vi "Homing RIO.vi"(7 "Offset Home 2 RCM":dbl[](array[numeric])=[0.0, 0.0, 0.0, 0.0], 8 "error in":errorcluster, 9 "Stage PID Cluster":T2={"Stage Z PID"={"Kp"=0.0005, "Kd"=0.001, "Ki"=0.0}, "Stage Y PID"={"Kp"=0.0003, "Kd"=0.01, "Ki"=0.0}, "Stage X PID"={"Kp"=0.0003, "Kd"=0.01, "Ki"=0.0}}, 10 "L1 to L4 PID Cluster":T1={"L1 PID Gains"={"Kp"=0.005, "Kd"=0.5, "Ki"=0.0005}, "L2 PID Gains"={"Kp"=0.01, "Kd"=1.0, "Ki"=0.005}, "L3 PID Gains"={"Kp"=0.05, "Kd"=1.0, "Ki"=0.0005}, "L4 PID Gains"={"Kp"=0.1, "Kd"=0.1, "Ki"=0.0005}}, 11 "FPGA VI Reference In":refnum<k20>) -> (0 "error out":errorcluster, 1 "Last Stage Posit":dbl[](array[numeric]), 2 "Last L1 to L4 Posit":dbl[](array[numeric]), 3 "FPGA VI Reference Out":refnum<k20>)   [LabVIEW 2016]
uses:
  <vilib>/Platform/TimedLoop/XDataNode/timing_clust.ctl
  <vilib>/Platform/TimedLoop/XDataNode/nitl_modes.ctl
  <vilib>/Platform/TimedLoop/XDataNode/wakeup.ctl
  Library/KevinLibraryAll/labview2010/kevLib2010/Simple Filters/kDelay.vi
  Global Variables.vi
  <vilib>/Utility/error.llb/Error Cluster From Error Code.vi
  <vilib>/rvi/errors/niLvFpgaAdjustHostInterfaceError.vi
  <vilib>/platform/TimedLoop/XDataNode/XDataNode.xnode
  <vilib>/rvi/interface/nirviReadWriteControl/nirviReadWriteControl.xnode
  FPGA Bitfiles/IRISSTrack_FPGATarget2_IRISSFPGAIORIO_4NTO9ubhv-c.lvbitx
  IRISS_FPGA_IO_RIO.vi
  <vilib>/Platform/TimedLoop/XDataNode/XDNodeRunTimeDep.lvlib
  Library/KevinLibraryAll/labview2010/kevLib2010.lvlib
  Library/KevinLibraryAll/labview2011/kevLib2011.lvlib
  Library/KevinLibraryAll/labview/KevLib01.lvlib
  Library/jmslib.lvlib
  NiFpgaLv.dll
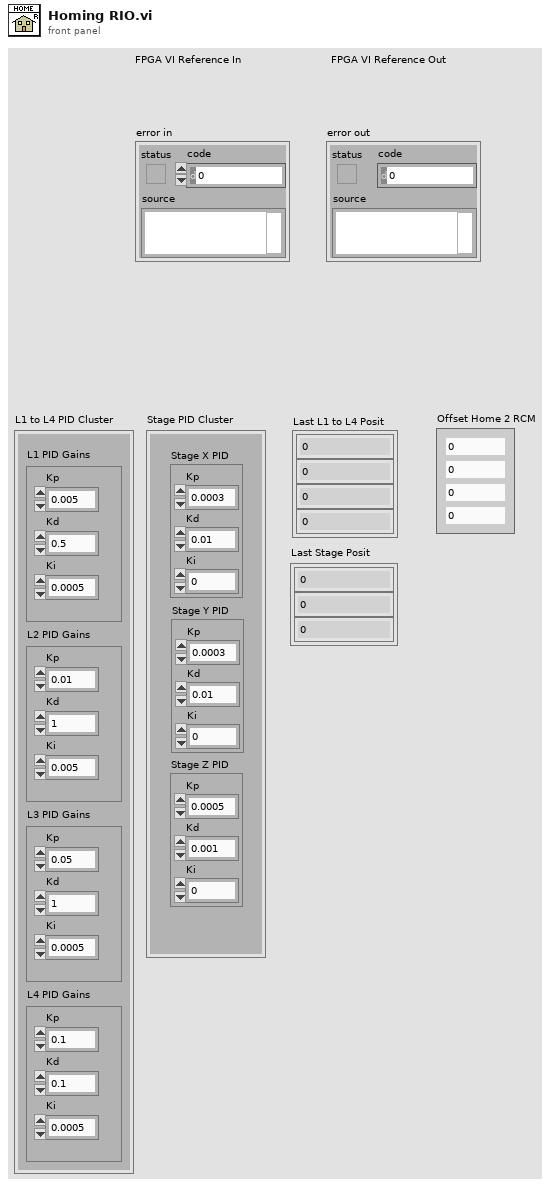
[diagram p1: front panel]
types:
  T1 = cluster{"L1 PID Gains":cluster{"Kp":dbl, "Kd":dbl, "Ki":dbl}, "L2 PID Gains":cluster{"Kp":dbl, "Kd":dbl, "Ki":dbl}, "L3 PID Gains":cluster{"Kp":dbl, "Kd":dbl, "Ki":dbl}, "L4 PID Gains":cluster{"Kp":dbl, "Kd":dbl, "Ki":dbl}}
  T2 = cluster{"Stage Z PID":cluster{"Kp":dbl, "Kd":dbl, "Ki":dbl}, "Stage Y PID":cluster{"Kp":dbl, "Kd":dbl, "Ki":dbl}, "Stage X PID":cluster{"Kp":dbl, "Kd":dbl, "Ki":dbl}}
  T3 = typedef "XDNodeRunTimeDep.lvlib/timing_clust.ctl" = cluster{"Expected End [f-1]":u64, "Actual End [f-1]":u64, "Finished Late? [f-1]":bool, "Expected End [i-1]":u64, "Actual End [i-1]":u64, "Finished Late? [i-1]":bool, "Expected Start [i]":u64, "Actual Start [i]":u64, "Expected Start [f]":u64, "Actual Start [f]":u64, "Source Name":string, "Structure Name":string, "Period":i64, "Deadline":i64, "Offset":i64, "Start":i64, "Priority":i32, "Timeout":i32, "Mode":T4, "Wakeup Reason":T5, "Error":errorcluster, "Source Type":string, "Secondary Source Type":string, "Global End Time":u64, "Global Start Time":u64, "Frame Duration":u64, "Iteration Duration":u64, "Assigned CPU":i32, "I/O Scan Engine Mode":u32}
  T4 = typedef "XDNodeRunTimeDep.lvlib/nitl_modes.ctl" = enum32{"No Change", "Process missed periods, maintain original phase", "Discard missed periods, maintain original phase", "Process missed periods, ignore original phase", "Discard missed periods, ignore original phase"}
  T5 = typedef "XDNodeRunTimeDep.lvlib/wakeup.ctl" = enum32{"Normal", "Aborted", "Asynchronous wakeup", "Timing source error", "Timed loop error", "Timeout"}
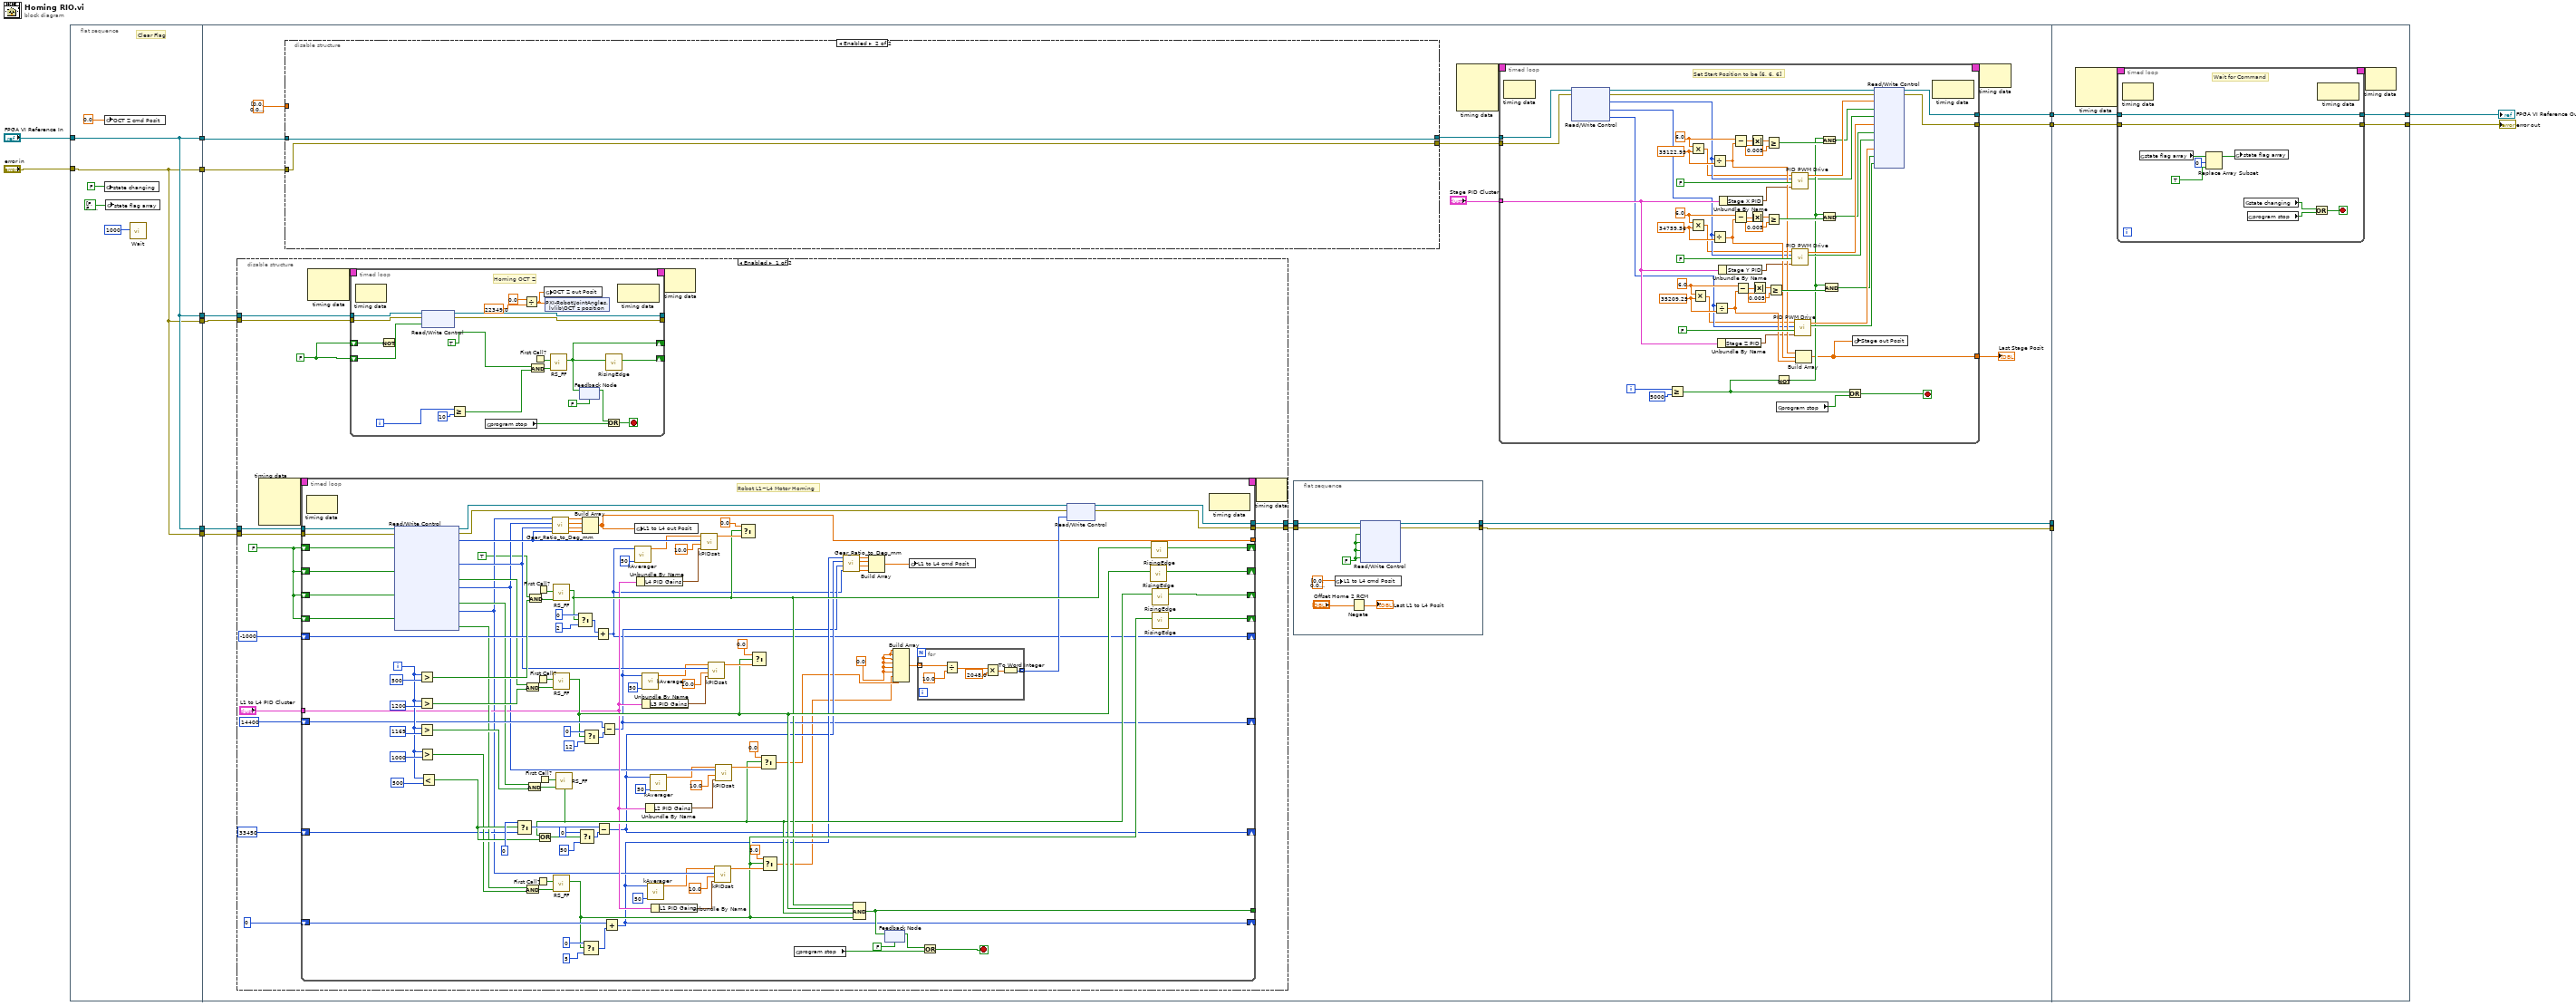
[diagram p0: block diagram]
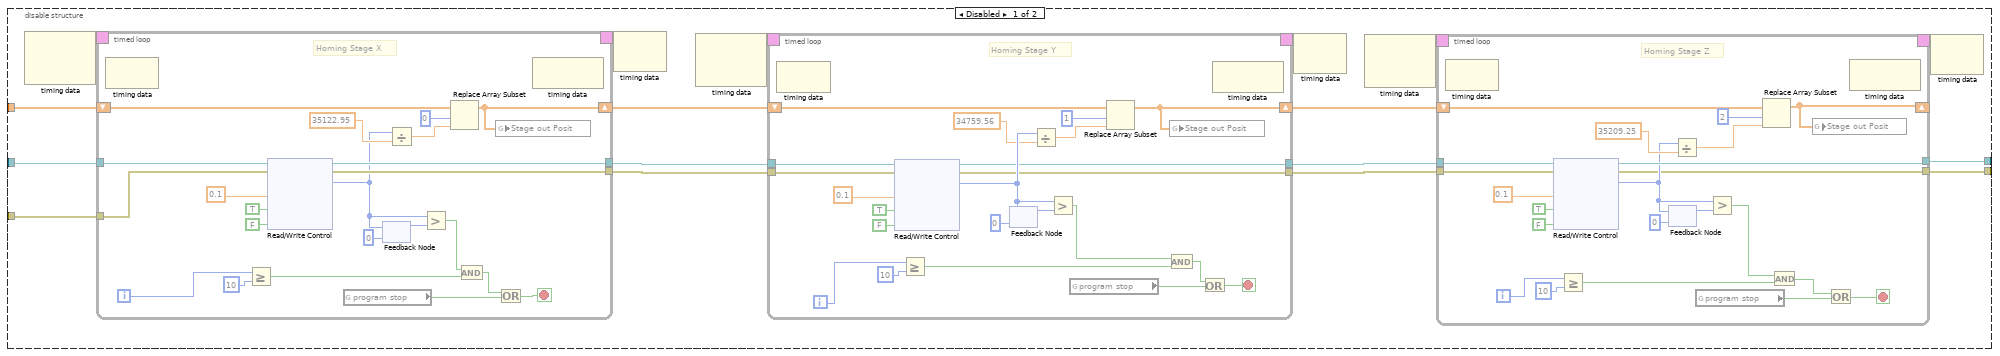
[diagram p3: hidden frame]
diagram:
  n1 = flat-sequence {
    tunnel: "FPGA VI Reference In" -> [w17]
    tunnel: "error in" -> [w16]
    tunnel: [w17] -> w14
    tunnel: [w17] -> w13
    tunnel: [w16] -> w12
    tunnel: [w16] -> w11
    tunnel: [w17] -> w6
    tunnel: [w16] -> w5
    tunnel: w14 -> [w37]
    tunnel: w13 -> [w36]
    tunnel: w12 -> [w35]
    tunnel: w11 -> [w34]
    tunnel: w6 -> [w33]
    tunnel: w5 -> [w32]
    tunnel: [w31] -> w4
    tunnel: [w30] -> w3
    tunnel: [w24] -> w2
    tunnel: [w23] -> w1
    tunnel: [w373] -> w8
    tunnel: [w372] -> w7
    tunnel: w4 -> [_]
    tunnel: w3 -> [_]
    tunnel: w2 -> [w371]
    tunnel: w1 -> [w370]
    frame #0 {
      # "Clear Flag"
      n2 = global write "Global Variables.vi" "OCT Z cmd Posit"(0.0) -> ()
      n3 = global write "Global Variables.vi" "state changing"(FALSE ("state changing")) -> ()
      n4 = global write "Global Variables.vi" "state flag array"(bool[] [FALSE, FALSE, FALSE, FALSE, FALSE, FALSE, FALSE, FALSE, FALSE] ("state flag array")) -> ()
      n5 = call "Wait"("Count(mSec)"=u32 1000 ("milliseconds to wait")) -> ()  [unwired: 1 out]
    }
    frame #1 {
      n6 = disable-structure shown="Enabled" {
        disable-tunnel: w36 -> [w52 _]
        disable-tunnel: w34 -> [w51 _]
        disable-tunnel: w33 -> [w50 _]
        disable-tunnel: w32 -> [w49 _]
        disable-tunnel: [w47 _] -> w22
        disable-tunnel: [w46 _] -> w21
        frame Enabled {
          w45 = FALSE ("Rising Edge")
          w48 = FALSE ("Rising Edge")
          n7 = node-c288() -> (w54:T3)  [unwired: 4 in]
          n8 = timed-loop {
            timing: w54 -> [_]
            timing-out: [_] -> w53
            tunnel: w52 -> [w169]
            tunnel: w51 -> [w168]
            shift-right: [w103] -> _
            shift-left: w45 -> [w167]
            shift-right: [w102] -> _
            shift-left: w45 -> [w166]
            shift-right: [w101] -> _
            shift-left: w45 -> [w165]
            shift-right: [w100] -> _
            shift-left: w45 -> [w164]
            shift-right: [w63] -> _
            shift-left: -1000 -> [w147]
            shift-right: [w64] -> _
            shift-left: 14400 -> [w139]
            shift-right: [w65] -> _
            shift-left: 33450 -> [w110]
            shift-right: [w66] -> _
            shift-left: 0 -> [w109]
            tunnel: [w104] -> _
            tunnel: [w89] -> w47
            tunnel: [w88] -> w46
            tunnel: "L1 to L4 PID Cluster" -> [w84]
            tunnel: [w62] -> _
            i -> [w149]
            stop <- w105 stop-if-true
            w57 = 0.0 ("element")
            # "Robot L1~L4 Motor Homing"
            n9 = node-c288() -> ()  [unwired: 1 in, 1 out]
            n10 = xnode "Read/Write Control"("FPGA VI Reference In"=w169, "error in"=w168, "Reset C1-4"=w167, "Reset C1-1"=w166, "Reset 3"=w165, "Reset 1"=w164) -> ("FPGA VI Reference Out"=w93:refnum<k20>, "error out"=w92:errorcluster, "32 bit Position C1-4"=w82:i32, "32 bit Position C1-1"=w81:i32, "Home L3"=w130:bool, "32 bit Position 3"=w80:i32, "Home L2"=w128:bool, "32 bit Position 1"=w79:i32, "Home L1"=w115:bool)  [unwired: 1 out]
            n11 = Greater?(x=w149, y=500) -> (0:w148:bool)
            n12 = Greater?(x=w149, y=1200) -> (0:w131:bool)
            n13 = Greater?(x=w149, y=1169) -> (0:w129:bool)
            n14 = Greater?(x=w149, y=1000) -> (0:w114:bool)
            n15 = Less?(x=w149, y=500) -> (x < y?=w121:bool)
            n16 = Select(t=0, s=w121, f=w110) -> (s? t:f=w126:i32)
            n17 = And(x=w130, y=w131) -> (x .and. y?=w140:bool)
            n18 = And(x=w115, y=w114) -> (x .and. y?=w116:bool)
            n19 = And(x=w128, y=w129) -> (x .and. y?=w133:bool)
            n20 = And(x=TRUE, y=w148) -> (x .and. y?=w160:bool)
            n21 = First Call?() -> (First Call?: T/F=w141:bool)
            n22 = First Call?() -> (First Call?: T/F=w117:bool)
            n23 = First Call?() -> (First Call?: T/F=w159:bool)
            n24 = First Call?() -> (First Call?: T/F=w132:bool)
            n25 = call "Gear_Ratio_to_Deg_mm.vi"("j4"=w82, "j3"=w81, "j2"=w80, "j1"=w79) -> ("theta 4"=w75:dbl, "theta 3"=w76:dbl, "theta 2"=w77:dbl, "theta 1"=w78:dbl)
            n26 = call "RS_FF.vi"("Set"=w160, "Reset"=w159) -> ("Result"=w97:bool)  [unwired: 9 in]
            n27 = call "RS_FF.vi"("Set"=w140, "Reset"=w141) -> ("Result"=w98:bool)  [unwired: 9 in]
            n28 = call "RS_FF.vi"("Set"=w116, "Reset"=w117) -> ("Result"=w99:bool)  [unwired: 9 in]
            n29 = call "RS_FF.vi"("Set"=w133, "Reset"=w132) -> ("Result"=w96:bool)  [unwired: 9 in]
            n30 = Or(x=w96, y=w121) -> (x .or. y?=w125:bool)
            n31 = Select(t=0, s=w97, f=2) -> (s? t:f=w161:i32)
            n32 = Select(t=0, s=w125, f=50) -> (s? t:f=w122:i32)
            n33 = Build Array(w78, w77, w76, w75) -> (w62:dbl[])
            n34 = Select(t=0, s=w99, f=5) -> (s? t:f=w120:i32)
            n35 = Select(t=0, s=w98, f=12) -> (s? t:f=w142:i32)
            n36 = Add(x=w161, y=w147) -> (x+y=w63:i32)
            n37 = Subtract(x=w126, y=w122) -> (x-y=w65:i32)
            n38 = Subtract(x=w139, y=w142) -> (x-y=w64:i32)
            n39 = Add(x=w109, y=w120) -> (x+y=w66:i32)
            n40 = call "kAverager.vi"("num avg"=50, "input"=w63) -> ("output"=w67:dbl)  [unwired: 9 in]
            n41 = global write "Global Variables.vi" "L1 to L4 out Posit"(w62) -> ()
            n42 = Unbundle By Name(w84) -> ("L4 PID Gains"=w87:cluster{"Kp":dbl, "Kd":dbl, "Ki":dbl})
            n43 = Unbundle By Name(w84) -> ("L3 PID Gains"=w86:cluster{"Kp":dbl, "Kd":dbl, "Ki":dbl})
            n44 = call "kAverager.vi"("num avg"=50, "input"=w64) -> ("output"=w68:dbl)  [unwired: 9 in]
            n45 = Unbundle By Name(w84) -> ("L2 PID Gains"=w85:cluster{"Kp":dbl, "Kd":dbl, "Ki":dbl})
            n46 = call "kAverager.vi"("num avg"=50, "input"=w66) -> ("output"=w70:dbl)  [unwired: 9 in]
            n47 = call "kAverager.vi"("num avg"=50, "input"=w65) -> ("output"=w69:dbl)  [unwired: 9 in]
            n48 = Unbundle By Name(w84) -> ("L1 PID Gains"=w83:cluster{"Kp":dbl, "Kd":dbl, "Ki":dbl})
            n49 = call "kPIDsat.vi"("PID Gains"=w87, "Sat Limit"=10.0, "Position"=w82, "Reference"=w67) -> ("Control"=w156:dbl)  [unwired: 7 in]
            n50 = call "kPIDsat.vi"("PID Gains"=w86, "Sat Limit"=10.0, "Position"=w81, "Reference"=w68) -> ("Control"=w137:dbl)  [unwired: 7 in]
            n51 = call "kPIDsat.vi"("PID Gains"=w83, "Sat Limit"=10.0, "Position"=w79, "Reference"=w70) -> ("Control"=w111:dbl)  [unwired: 7 in]
            n52 = call "kPIDsat.vi"("PID Gains"=w85, "Sat Limit"=10.0, "Position"=w80, "Reference"=w69) -> ("Control"=w136:dbl)  [unwired: 7 in]
            n53 = Select(t=0.0, s=w97, f=w156) -> ()  [unwired: 1 out]
            n54 = Select(t=0.0 ("element"), s=w98, f=w137) -> ()  [unwired: 1 out]
            n55 = Select(t=0.0 ("element"), s=w96, f=w136) -> (s? t:f=w59:dbl)
            n56 = Select(t=3.0 ("element"), s=w99, f=w111) -> (s? t:f=w58:dbl)
            n57 = global read "Global Variables.vi" "program stop"() -> (w106:bool)
            n58 = call "Gear_Ratio_to_Deg_mm.vi"("j4"=w63, "j3"=w64, "j2"=w65, "j1"=w66) -> ("theta 4"=w71:dbl, "theta 3"=w72:dbl, "theta 2"=w73:dbl, "theta 1"=w74:dbl)
            n59 = Compound Arithmetic op=AND(w97, w98, w96, w99) -> (w104:bool)
            n60 = Build Array(w74, w73, w72, w71) -> (w61:dbl[])
            n61 = feedback #1(FALSE) -> (w107:bool)
            n62 = feedback-in #1(w104) -> ()
            n63 = Build Array(w57, w57, w57, w57, w57, w57, w58, w59) -> (w95:dbl[])
            n64 = global write "Global Variables.vi" "L1 to L4 cmd Posit"(w61) -> ()
            n65 = for {
              tunnel: [w173] -> w94 mode=indexing
              tunnel: w95 -> [w172] mode=indexing
              n66 = Divide(x=w172, y=10.0) -> (x/y=w175:dbl)
              n67 = Multiply(x=w175, y=2048.0) -> (x*y=w174:dbl)
              n68 = To Word Integer(number=w174) -> (16bit integer=w173:i16)
            }
            n69 = Or(x=w107, y=w106) -> (x .or. y?=w105:bool)
            n70 = xnode "Read/Write Control"("FPGA VI Reference In"=w93, "error in"=w92, "AO"=w94) -> ("FPGA VI Reference Out"=w89:refnum<k20>, "error out"=w88:errorcluster)
            n71 = call "RisingEdge.vi"("Signal In"=w98) -> ("Rising Edge"=w102:bool)  [unwired: 10 in]
            n72 = call "RisingEdge.vi"("Signal In"=w97) -> ("Rising Edge"=w103:bool)  [unwired: 10 in]
            n73 = call "RisingEdge.vi"("Signal In"=w96) -> ("Rising Edge"=w101:bool)  [unwired: 10 in]
            n74 = call "RisingEdge.vi"("Signal In"=w99) -> ("Rising Edge"=w100:bool)  [unwired: 10 in]
            n75 = node-c288() -> ()  [unwired: 1 in, 1 out]
          }
          n76 = node-c288() -> (w56:T3)  [unwired: 2 in]
          n77 = timed-loop {
            timing: w56 -> [_]
            timing-out: [_] -> w55
            tunnel: w50 -> [w197]
            tunnel: w49 -> [w196]
            tunnel: [w195] -> _
            tunnel: [w194] -> _
            shift-right: [w190] -> _
            shift-left: w48 -> [w191]
            shift-right: [w186] -> _
            shift-left: w48 -> [w184]
            i -> [w198]
            stop <- w192 stop-if-true
            # "Homing OCT Z"
            n78 = node-c288() -> ()  [unwired: 1 in, 1 out]
            n79 = Not(x=w184) -> ()  [unwired: 1 out]
            n80 = xnode "Read/Write Control"("FPGA VI Reference In"=w197, "error in"=w196, "Reset 14"=w191) -> ("FPGA VI Reference Out"=w195:refnum<k20>, "error out"=w194:errorcluster)
            n81 = Greater Or Equal?(x=w198, y=10) -> (x >= y?=w200:bool)
            n82 = global read "Global Variables.vi" "program stop"() -> (w193:bool)
            n83 = Divide(x=0.0, y=22349.0) -> (x/y=w182:dbl)
            n84 = And(x=TRUE, y=w200) -> (x .and. y?=w188:bool)
            n85 = First Call?() -> (First Call?: T/F=w189:bool)
            n86 = global write "Global Variables.vi" "OCT Z out Posit"(w182) -> ()
            n87 = shared-variable "PXI-Robot\\JointAngles.lvlib\\OCT z position"(w182) -> ()  [unwired: 1 in, 1 out]
            n88 = call "RS_FF.vi"("Set"=w188, "Reset"=w189) -> ("Result"=w186:bool)  [unwired: 9 in]
            n89 = feedback #2(FALSE) -> (w185:bool)
            n90 = feedback-in #2(w186) -> ()
            n91 = call "RisingEdge.vi"("Signal In"=w186) -> ("Rising Edge"=w190:bool)  [unwired: 10 in]
            n92 = Or(x=w185, y=w193) -> (x .or. y?=w192:bool)
            n93 = node-c288() -> ()  [unwired: 1 in, 1 out]
          }
          n94 = node-c288(w55) -> ()  [unwired: 1 out]
          n95 = node-c288(w53) -> ()  [unwired: 1 out]
        }
        frame Disabled {
        }
      }
      n96 = disable-structure shown="Enabled" {
        disable-tunnel: [w215 w301] -> w39
        disable-tunnel: [w214 w300] -> w38
        disable-tunnel: w37 -> [w213 w301]
        disable-tunnel: w35 -> [w212 w300]
        disable-tunnel: dbl[] [0.0, 0.0, 0.0] ("Stage Posit Array") -> [w205 _]
        frame Disabled {
          n97 = node-c288() -> (w217:T3)  [unwired: 2 in]
          n98 = timed-loop {
            timing: w217 -> [_]
            timing-out: [_] -> w216
            tunnel: w213 -> [w233]
            tunnel: w212 -> [w232]
            tunnel: [w231] -> w208
            tunnel: [w230] -> w207
            shift-right: [w222] -> w206
            shift-left: w205 -> [w224]
            i -> [w234]
            stop <- w227 stop-if-true
            # "Homing Stage X"
            n99 = node-c288() -> ()  [unwired: 1 in, 1 out]
            n100 = Greater Or Equal?(x=w234, y=10) -> (x >= y?=w243:bool)
            n101 = xnode "Read/Write Control"("FPGA VI Reference In"=w233, "error in"=w232, "X DC"=0.1 ("y"), "INHB X"=TRUE ("INHB Y"), "DIR X"=FALSE ("INHB Y")) -> ("FPGA VI Reference Out"=w231:refnum<k20>, "error out"=w230:errorcluster, "Position X"=w223:i32)
            n102 = global read "Global Variables.vi" "program stop"() -> (w229:bool)
            n103 = feedback #3(0 ("Position Y")) -> (w240:i32)
            n104 = feedback-in #3(w223) -> ()
            n105 = Divide(x=w223, y=35122.95) -> (x/y=w225:dbl)
            n106 = Greater?(x=w223, y=w240) -> (0:w241:bool)
            n107 = Replace Array Subset(array=w224, new element=w225, index=0) -> (w222:dbl[])
            n108 = And(x=w241, y=w243) -> (x .and. y?=w228:bool)
            n109 = global write "Global Variables.vi" "Stage out Posit"(w222) -> ()
            n110 = Or(x=w228, y=w229) -> (x .or. y?=w227:bool)
            n111 = node-c288() -> ()  [unwired: 1 in, 1 out]
          }
          n112 = node-c288(w216) -> ()  [unwired: 1 out]
          n113 = node-c288() -> (w219:T3)  [unwired: 2 in]
          n114 = timed-loop {
            timing: w219 -> [_]
            timing-out: [_] -> w218
            tunnel: w208 -> [w258]
            tunnel: w207 -> [w259]
            tunnel: [w256] -> w211
            tunnel: [w255] -> w210
            shift-right: [w248] -> w209
            shift-left: w206 -> [w249]
            i -> [w257]
            stop <- w254 stop-if-true
            # "Homing Stage Y"
            n115 = node-c288() -> ()  [unwired: 1 in, 1 out]
            n116 = xnode "Read/Write Control"("FPGA VI Reference In"=w258, "error in"=w259, "Y DC"=0.1 ("y"), "INHB Y"=TRUE, "DIR Y"=FALSE ("INHB Y")) -> ("FPGA VI Reference Out"=w256:refnum<k20>, "error out"=w255:errorcluster, "Position Y"=w266:i32)
            n117 = Greater Or Equal?(x=w257, y=10) -> (x >= y?=w269:bool)
            n118 = feedback #4(0 ("Position Y")) -> (w265:i32)
            n119 = feedback-in #4(w266) -> ()
            n120 = Divide(x=w266, y=34759.56) -> (x/y=w250:dbl)
            n121 = Greater?(x=w266, y=w265) -> (0:w267:bool)
            n122 = global read "Global Variables.vi" "program stop"() -> (w252:bool)
            n123 = Replace Array Subset(array=w249, new element=w250, index=1) -> (w248:dbl[])
            n124 = And(x=w267, y=w269) -> (x .and. y?=w253:bool)
            n125 = global write "Global Variables.vi" "Stage out Posit"(w248) -> ()
            n126 = Or(x=w253, y=w252) -> (x .or. y?=w254:bool)
            n127 = node-c288() -> ()  [unwired: 1 in, 1 out]
          }
          n128 = node-c288(w218) -> ()  [unwired: 1 out]
          n129 = node-c288() -> (w221:T3)  [unwired: 2 in]
          n130 = timed-loop {
            timing: w221 -> [_]
            timing-out: [_] -> w220
            tunnel: w211 -> [w295]
            tunnel: [w294] -> w215
            tunnel: w210 -> [w282]
            tunnel: [w281] -> w214
            shift-right: [w274] -> _
            shift-left: w209 -> [w275]
            i -> [w285]
            stop <- w279 stop-if-true
            # "Homing Stage Z"
            n131 = node-c288() -> ()  [unwired: 1 in, 1 out]
            n132 = xnode "Read/Write Control"("FPGA VI Reference In"=w295, "error in"=w282, "Z DC"=0.1 ("y"), "INHB Z"=TRUE ("INHB Y"), "DIR Z"=FALSE ("INHB Y")) -> ("FPGA VI Reference Out"=w294:refnum<k20>, "error out"=w281:errorcluster, "Position Z"=w287:i32)
            n133 = Greater Or Equal?(x=w285, y=10) -> (x >= y?=w283:bool)
            n134 = feedback-in #5(w287) -> ()
            n135 = feedback #5(0 ("Position Y")) -> (w288:i32)
            n136 = Divide(x=w287, y=35209.25) -> (x/y=w276:dbl)
            n137 = global read "Global Variables.vi" "program stop"() -> (w280:bool)
            n138 = Greater?(x=w287, y=w288) -> (0:w286:bool)
            n139 = Replace Array Subset(array=w275, new element=w276, index=2) -> (w274:dbl[])
            n140 = And(x=w286, y=w283) -> (x .and. y?=w278:bool)
            n141 = global write "Global Variables.vi" "Stage out Posit"(w274) -> ()
            n142 = Or(x=w278, y=w280) -> (x .or. y?=w279:bool)
            n143 = node-c288() -> ()  [unwired: 1 in, 1 out]
          }
          n144 = node-c288(w220) -> ()  [unwired: 1 out]
        }
        frame Enabled {
        }
      }
      n145 = flat-sequence {
        tunnel: w22 -> [w308]
        tunnel: w21 -> [w307]
        tunnel: [w303] -> w31
        tunnel: [w302] -> w30
        frame #0 {
          w309 = FALSE ("Reset 1")
          n146 = global write "Global Variables.vi" "L1 to L4 cmd Posit"(dbl[] [0.0, 0.0, 0.0, 0.0] ("L1 to L4 cmd Posit")) -> ()
          n147 = Negate(x="Offset Home 2 RCM") -> (-x=→"Last L1 to L4 Posit":dbl[])
          n148 = xnode "Read/Write Control"("FPGA VI Reference In"=w308, "error in"=w307, "Reset C1-4"=w309, "Reset C1-1"=w309, "Reset 3"=w309, "Reset 1"=w309) -> ("FPGA VI Reference Out"=w303:refnum<k20>, "error out"=w302:errorcluster)
        }
      }
      n149 = node-c288() -> (w29:T3)  [unwired: 4 in]
      n150 = timed-loop {
        timing: w29 -> [_]
        timing-out: [_] -> w28
        tunnel: w39 -> [w330]
        tunnel: w38 -> [w331]
        tunnel: "Stage PID Cluster" -> [w339]
        tunnel: [w312] -> w26
        tunnel: [w311] -> w24
        tunnel: [w310] -> w23
        i -> [w365]
        stop <- w329 stop-if-true
        w342 = 6.0 ("y")
        w345 = 35209.25 ("y")
        w356 = 6.0 ("y")
        w353 = 34759.56 ("y")
        w357 = 6.0 ("y")
        w360 = 35122.95 ("y")
        # "Set Start Position to be [6, 6, 6]"
        n151 = node-c288() -> ()  [unwired: 1 in, 1 out]
        n152 = xnode "Read/Write Control"("FPGA VI Reference In"=w330, "error in"=w331) -> ("FPGA VI Reference Out"=w333:refnum<k20>, "error out"=w332:errorcluster, "Position X"=w328:i32, "Position Y"=w327:i32, "Position Z"=w326:i32)
        n153 = Greater Or Equal?(x=w365, y=5000) -> (x >= y?=w318:bool)
        n154 = Multiply(x=w357, y=w360) -> (x*y=w325:dbl)
        n155 = Multiply(x=w356, y=w353) -> (x*y=w324:dbl)
        n156 = Multiply(x=w342, y=w345) -> (x*y=w323:dbl)
        n157 = Divide(x=w328, y=w360) -> (x/y=w338:dbl)
        n158 = Divide(x=w327, y=w353) -> (x/y=w337:dbl)
        n159 = Divide(x=w326, y=w345) -> (x/y=w336:dbl)
        n160 = Unbundle By Name(w339) -> ("Stage Z PID"=w334:cluster{"Kp":dbl, "Kd":dbl, "Ki":dbl})
        n161 = Unbundle By Name(w339) -> ("Stage Y PID"=w335:cluster{"Kp":dbl, "Kd":dbl, "Ki":dbl})
        n162 = Unbundle By Name(w339) -> ("Stage X PID"=w319:cluster{"Kp":dbl, "Kd":dbl, "Ki":dbl})
        n163 = Subtract(x=w357, y=w338) -> (x-y=w361:dbl)
        n164 = Subtract(x=w356, y=w337) -> (x-y=w352:dbl)
        n165 = Subtract(x=w342, y=w336) -> (x-y=w346:dbl)
        n166 = Absolute Value(x=w361) -> (abs(x)=w362:dbl)
        n167 = Absolute Value(x=w352) -> (abs(x)=w351:dbl)
        n168 = Absolute Value(x=w346) -> (abs(x)=w347:dbl)
        n169 = Greater Or Equal?(x=w362, y=0.005) -> (x >= y?=w358:bool)
        n170 = Greater Or Equal?(x=w351, y=0.005) -> (x >= y?=w355:bool)
        n171 = Greater Or Equal?(x=w347, y=0.005) -> (x >= y?=w343:bool)
        n172 = Not(x=w318) -> (.not. x?=w317:bool)
        n173 = global read "Global Variables.vi" "program stop"() -> (w340:bool)
        n174 = call "PID PWM Drive.vi"("PID Gains"=w319, "Reverse Motor?"=FALSE, "Encoder Position"=w328, "Reference"=w325) -> ("Direction"=w315:bool, "Duty Cycle"=w322:dbl)  [unwired: 5 in, 1 out]
        n175 = call "PID PWM Drive.vi"("PID Gains"=w335, "Reverse Motor?"=FALSE, "Encoder Position"=w327, "Reference"=w324) -> ("Direction"=w349:bool, "Duty Cycle"=w321:dbl)  [unwired: 5 in, 1 out]
        n176 = call "PID PWM Drive.vi"("PID Gains"=w334, "Reverse Motor?"=FALSE, "Encoder Position"=w326, "Reference"=w323) -> ("Direction"=w341:bool, "Duty Cycle"=w320:dbl)  [unwired: 5 in, 1 out]
        n177 = Build Array(w338, w337, w336) -> (w312:dbl[])
        n178 = And(x=w317, y=w358) -> (x .and. y?=w316:bool)
        n179 = And(x=w317, y=w355) -> (x .and. y?=w314:bool)
        n180 = And(x=w317, y=w343) -> (x .and. y?=w313:bool)
        n181 = Or(x=w318, y=w340) -> (x .or. y?=w329:bool)
        n182 = global write "Global Variables.vi" "Stage out Posit"(w312) -> ()
        n183 = xnode "Read/Write Control"("FPGA VI Reference In"=w333, "error in"=w332, "X DC"=w322, "INHB X"=w316, "DIR X"=w315, "Y DC"=w321, "INHB Y"=w314, "DIR Y"=w349, "Z DC"=w320, "INHB Z"=w313, "DIR Z"=w341) -> ("FPGA VI Reference Out"=w311:refnum<k20>, "error out"=w310:errorcluster)
        n184 = node-c288() -> ()  [unwired: 1 in, 1 out]
      }
      "Last Stage Posit" <- w26
      n185 = node-c288(w28) -> ()  [unwired: 1 out]
    }
    frame #2 {
      n186 = node-c288() -> (w375:T3)  [unwired: 3 in]
      n187 = timed-loop {
        timing: w375 -> [_]
        timing-out: [_] -> w374
        tunnel: w371 -> [w378]
        tunnel: [w378] -> w373
        tunnel: [w377] -> w372
        tunnel: w370 -> [w377]
        stop <- w376 stop-if-true
        # "Wait for Command"
        n188 = node-c288() -> ()  [unwired: 1 in, 1 out]
        n189 = global read "Global Variables.vi" "state flag array"() -> (w382:bool[])
        n190 = Replace Array Subset(array=w382, new element=TRUE ("new element/subarray"), index=0) -> (w381:bool[])
        n191 = global write "Global Variables.vi" "state flag array"(w381) -> ()
        n192 = global read "Global Variables.vi" "state changing"() -> (w384:bool)
        n193 = global read "Global Variables.vi" "program stop"() -> (w383:bool)
        n194 = Or(x=w384, y=w383) -> (x .or. y?=w376:bool)
        n195 = node-c288() -> ()  [unwired: 1 in, 1 out]
      }
      n196 = node-c288(w374) -> ()  [unwired: 1 out]
    }
  }
  "FPGA VI Reference Out" <- w8
  "error out" <- w7
